vi "WriteValueNames.vi"(8 "error in (no error)":errorcluster, 10 "ValueNames":cluster{refnum<class "CodeElement.lvclass">[]}[](array[cluster]), 11 "object in":refnum<class "SwitchCaseElement.lvclass">) -> (0 "error out":errorcluster, 3 "object out":refnum<class "SwitchCaseElement.lvclass">)   [LabVIEW 2017, in "SwitchCaseElement.lvclass"]
uses:
  SwitchCaseElement.lvclass
  Base/CodeElement.lvclass
  SwitchCaseElement.lvclass/SwitchCaseElement.ctl
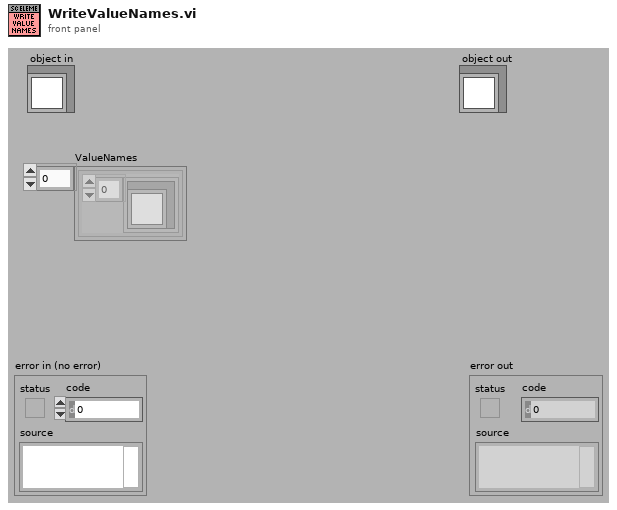
[diagram p1: front panel]
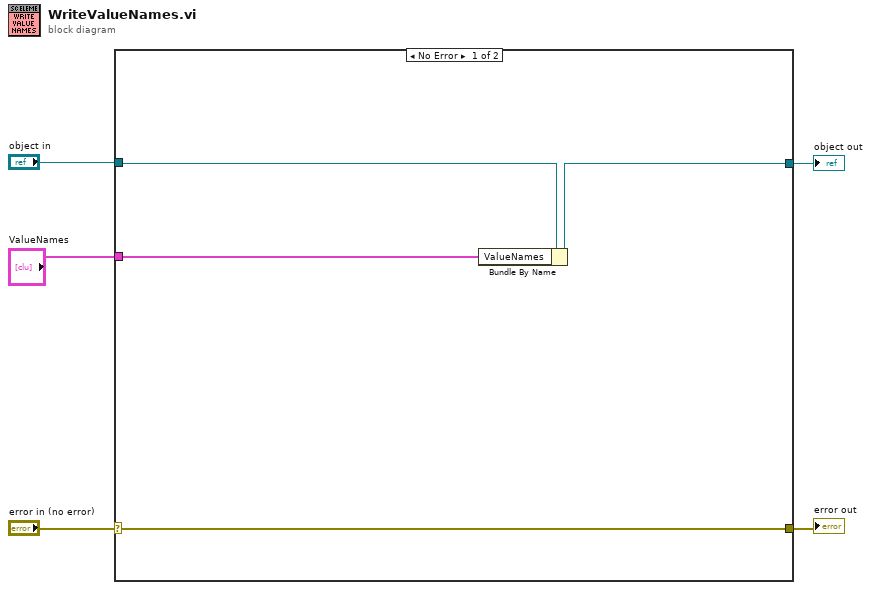
[diagram p0: block diagram]
diagram:
  n1 = case shown="No Error" "error in (no error)" {
    selector: "error in (no error)" -> [w8 w11]
    tunnel: [w8 w11] -> w4
    tunnel: [w6 w10] -> w2
    tunnel: "object in" -> [w7 w10]
    tunnel: "ValueNames" -> [w9 _]
    frame No Error {
      n2 = Bundle By Name(cluster=w7, "ValueNames"=w9) -> (w6:refnum<class "SwitchCaseElement.lvclass">)
    }
    frame Error {
    }
  }
  "error out" <- w4
  "object out" <- w2
